vi "Document.vi"(5 "EndTime":timestamp, 7 "StartTime":timestamp, 8 "error in (no error)":errorcluster, 11 "Characteristic in":refnum<class "Document.lvclass">) -> (0 "error out":errorcluster, 3 "Passed":bool)   [LabVIEW 2020]
uses:
  ProligentResultProcessor/Model/Document/Document.lvclass
  ProligentResultProcessor/Model/Document/SetDescription.vi
  ProligentResultProcessor/Model/Document/SetFileName.vi
  ProligentResultProcessor/Model/Document/SetIdentifier.vi
  ProligentResultProcessor/Model/Document/SetName.vi
  ProligentResultProcessor/Model/Document/GetDescription.vi
  ProligentResultProcessor/Model/Document/GetFileName.vi
  ProligentResultProcessor/Model/Document/GetIdentifier.vi
  ProligentResultProcessor/Model/Document/GetName.vi
  ProligentResultProcessor/Model/Document/GetCustomData.vi
  ProligentResultProcessor/Model/CustomData/CustomData.lvclass
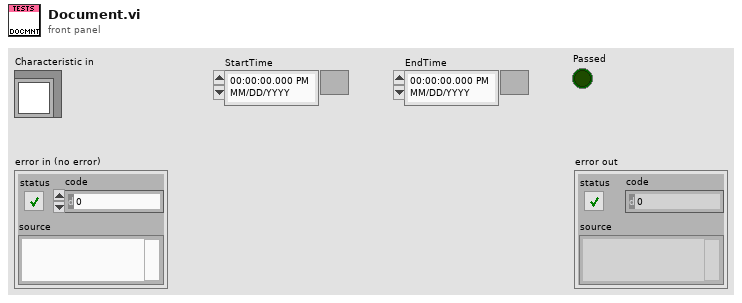
[diagram p1: front panel]
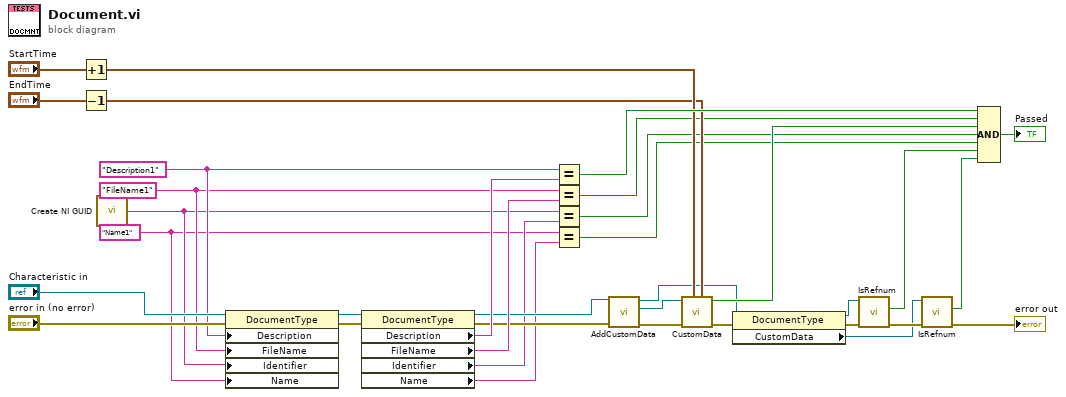
[diagram p0: block diagram]
diagram:
  w1 = "Name1"
  w28 = "FileName1"
  w30 = "Description1"
  n1 = Increment(x="StartTime") -> (x+1=w20:timestamp)
  n2 = Decrement(x="EndTime") -> (x-1=w19:timestamp)
  n3 = call <vilib>:"Create NI GUID.vi"() -> ("NI GUID"=w2:string)
  n4 = property class="DocumentType"(reference="Characteristic in", error in="error in (no error)", "Description"=w30, "FileName"=w28, "Identifier"=w2, "Name"=w1) -> (reference out=w33:refnum<class "Document.lvclass">, error out=w32:errorcluster)
  n5 = property class="DocumentType"(reference=w33, error in=w32) -> (reference out=w26:refnum<class "Document.lvclass">, error out=w27:errorcluster, "Description"=w31:string, "FileName"=w29:string, "Identifier"=w6:string, "Name"=w5:string)
  n6 = Equal?(x=w30, y=w31) -> (x = y?=w25:bool)
  n7 = Equal?(x=w28, y=w29) -> (x = y?=w7:bool)
  n8 = Equal?(x=w2, y=w6) -> (x = y?=w4:bool)
  n9 = Equal?(x=w1, y=w5) -> (x = y?=w3:bool)
  n10 = call "AddCustomData.vi"("error in"=w27, "Document in"=w26) -> ("error out"=w23:errorcluster, "CustomData"=w24:refnum<class "CustomData.lvclass">, "Document out"=w14:refnum<class "Document.lvclass">)  [unwired: 7 in]
  n11 = call "CustomData.vi"("EndTime"=w19, "StartTime"=w20, "error in"=w23, "CustomData"=w24) -> ("error out"=w17:errorcluster, "Passed"=w18:bool)  [unwired: 6 in]
  n12 = property class="DocumentType"(reference=w14, error in=w17) -> (reference out=w13:refnum<class "Document.lvclass">, error out=w15:errorcluster, "CustomData"=w10:refnum<class "CustomData.lvclass">)
  n13 = call "IsRefnum.vi"("error in"=w15, "Document in"=w13) -> ("error out"=w11:errorcluster, "IsRefnum"=w16:bool)  [unwired: 7 in, 1 out]
  n14 = call "IsRefnum.vi"("error in"=w11, "CustomDataType in"=w10) -> ("error out"=→"error out":errorcluster, "IsRefnum"=w9:bool)  [unwired: 7 in, 1 out]
  n15 = Compound Arithmetic op=AND(w25, w7, w18, w4, w3, w16, w9) -> (→"Passed":bool)
